vi "Init Event materiel Start.vi"(8 "error in (no error)":errorcluster caption="entrée d'erreur (pas d'erreur)", 9 "Event start test":refnum<user-event>, 10 "Part Number PCBA":string(combo), 11 "Type Product":string(combo)) -> (0 "error out":errorcluster caption="sortie d'erreur")   [LabVIEW 2020]
uses:
  Class/Instrument/Instrument (Default)/Class Instrument (Default).lvclass
  TypeDef/Variable Printable.ctl
  Class/Core/Actors/Actor_EventStart/Actor_EventStart/Actor_EventStart.lvclass
  C:/Program Files (x86)/National Instruments/LabVIEW 2020/vi.lib/ActorFramework/Actor/Actor.lvclass
  Class/Core/Actors/Actor_EventStart/Actor_EventStart Messages/Message Show_GUI/Message Show_GUI.lvclass/Message Show_GUI.ctl
  <vilib>/ActorFramework/Message Enqueuer/Message Enqueuer.lvclass/Message Enqueuer.ctl
  Class/Core/Actors/Actor_EventStart/Actor_EventStart Messages/Message Parameter/Message Parameter.lvclass/Message Parameter.ctl
  <vilib>/ActorFramework/Message Enqueuer/Enqueue.vi
  Class/Core/Actors/Actor_EventStart/Actor_EventStart Messages/Message Show_GUI/Message Show_GUI.lvclass
  C:/Program Files (x86)/National Instruments/LabVIEW 2020/vi.lib/ActorFramework/Message/Message.lvclass
  Class/Core/Actors/Actor_EventStart/Actor_EventStart Messages/Message Parameter/Message Parameter.lvclass
  <vilib>/Utility/config.llb/Read Key (String).vi
  <vilib>/ActorFramework/Message Priority Queue/Priority Enqueue.vi
  Library Commun.lvlib
  <vilib>/Utility/config.llb/NI_LVConfig.lvlib
  <vilib>/ActorFramework/Actor/Actor.lvclass
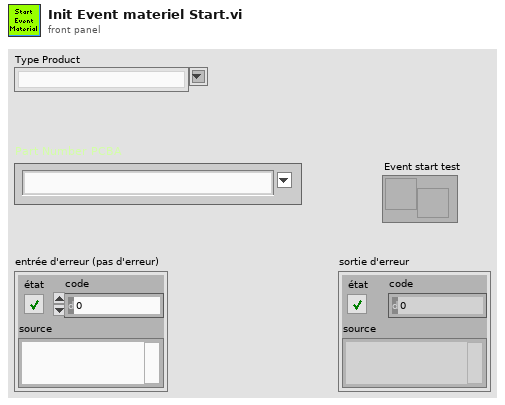
[diagram p1: front panel]
types:
  T1 = enum16{"Add Instr", "Remove Instr", "List Instr", "Get Instr Class", "Get Instr obj", "Save Insrt obj", "Modify Insrt obj", "Init"}
  T2 = enum16{"Not Use", "Wait Event", "Test in progress", "Test Stopped"}
  T3 = typedef "Variable Printable.ctl" = string
  T4 = enum16{"Get Variable", "Get All Variables", "Set Variable", "Delete Variable", "Delete All Variable"}
  T5 = cluster{"Class Event":string, "Awaited Event":string, "Instruments":refnum<class "Class Instrument (Default).lvclass">, "Event Start BP":refnum<user-event>}
  T6 = enum16{"Init", "Add Actor", "Delete Actor", "Get Actor Queue", "Get Log Actor Queue", "List all actors"}
  T7 = typedef "NI_LVConfig.lvlib/Config Data RefNum.ctl" = refnum<k1>
  T8 = cluster{"Name":string, "Instrument":refnum<class "Class Instrument (Default).lvclass">, "Close After Autotest":bool}[]
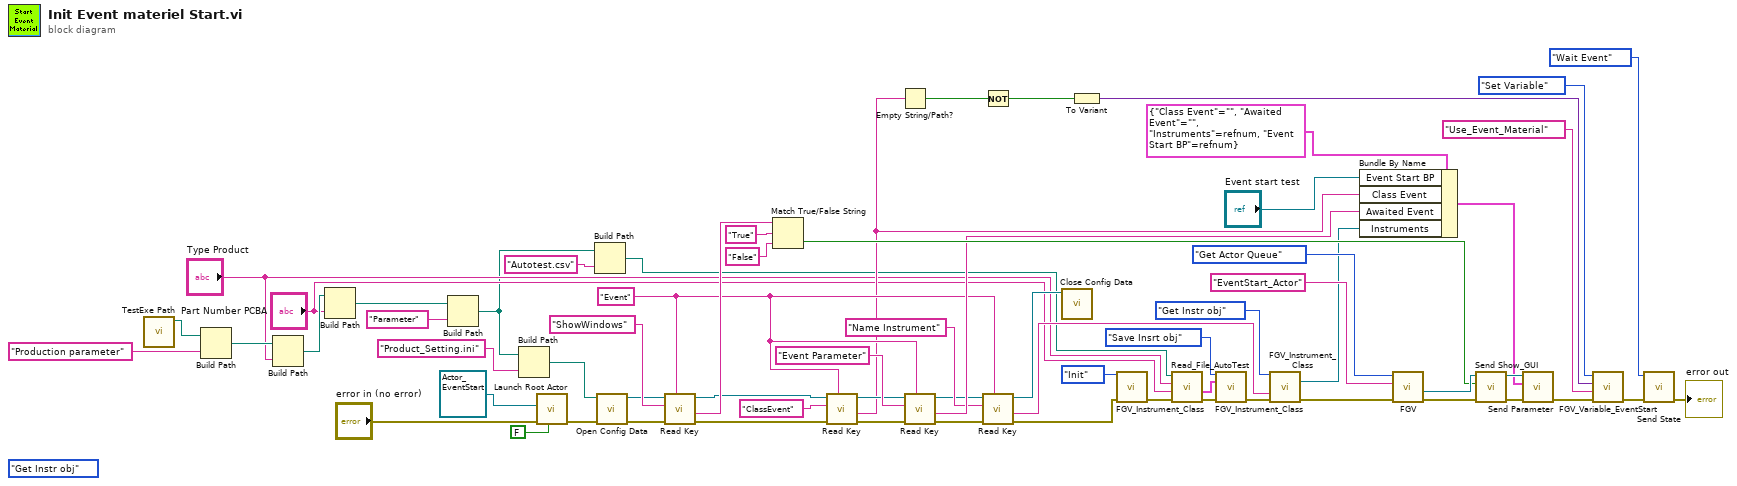
[diagram p0: block diagram]
diagram:
  (unwired) T1."Get Instr obj" ("Action")
  w39 = "Event" ("nom ou chemin relatif")
  n1 = call "TestExe Path.vi"() -> ("Chemin Actuel"=w36:path)  [unwired: 9 in, 2 out]
  n2 = Build Path(base path=w36, name or relative path="Production parameter" ("nom ou chemin relatif")) -> (appended path=w58:path)
  n3 = Build Path(base path=w58, name or relative path="Type Product") -> (appended path=w57:path)
  n4 = Build Path(base path=w57, name or relative path="Part Number PCBA") -> (appended path=w56:path)
  n5 = Build Path(base path=w56, name or relative path="Parameter" ("nom ou chemin relatif")) -> (appended path=w9:path)
  n6 = Build Path(base path=w9, name or relative path="Product_Setting.ini" ("nom ou chemin relatif")) -> (appended path=w14:path)
  n7 = call <vilib>:"Launch Root Actor.vi"("Open Actor Core front panel? (F)"=FALSE, "error in (no error)"="error in (no error)", "Actor"=refnum<class "Actor_EventStart.lvclass"> refnum ("Library Sequencer.lvlib:Actor_EventStart.lvlib:Actor_EventStart.lvclass")) -> ("error out"=w4:errorcluster)  [unwired: 7 in, 1 out]
  n8 = Build Path(base path=w9, name or relative path="Autotest.csv" ("nom ou chemin relatif")) -> (appended path=w19:path)
  n9 = call <vilib>:"Open Config Data.vi"("error in (no error)"=w4, "configuration file path"=w14) -> ("error out"=w53:errorcluster, "refnum"=w52:T7)  [unwired: 7 in, 1 out]
  n10 = call-poly <vilib>:"Read Key.vi"("section"=w39, "error in (no error)"=w53, "key"="ShowWindows", "refnum"=w52) -> ("error out"=w47:errorcluster, "value"=w49:string, "refnum out"=w31:T7)  [unwired: 4 in, 1 out]
  n11 = Match True/False String(2:"False" ("chaîne faux"), 3:"True" ("chaîne vrai"), 4:w49) -> (0:w48:bool)  [unwired: 1 out]
  n12 = call-poly <vilib>:"Read Key.vi"("section"=w39, "error in (no error)"=w47, "key"="ClassEvent", "refnum"=w31) -> ("error out"=w41:errorcluster, "value"=w25:string, "refnum out"=w30:T7)  [unwired: 4 in, 1 out]
  n13 = Empty String/Path?(string/path=w25) -> (empty?=w24:bool)
  n14 = call-poly <vilib>:"Read Key.vi"("section"=w39, "error in (no error)"=w41, "key"="Event Parameter", "refnum"=w30) -> ("error out"=w40:errorcluster, "value"=w43:string, "refnum out"=w29:T7)  [unwired: 4 in, 1 out]
  n15 = Not(x=w24) -> (.not. x?=w20:bool)
  n16 = call-poly <vilib>:"Read Key.vi"("section"=w39, "error in (no error)"=w40, "key"="Name Instrument", "refnum"=w29) -> ("error out"=w13:errorcluster, "value"=w34:string, "refnum out"=w37:T7)  [unwired: 4 in, 1 out]
  n17 = call <vilib>:"Close Config Data.vi"("refnum"=w37) -> ()  [unwired: 9 in, 2 out]
  n18 = To Variant(anything=w20) -> (Variant=w26:variant)
  n19 = call "FGV_Instrument_Class.vi"("Action"=T1."Init", "error in (no error)"=w13) -> ("error out"=w15:errorcluster)  [unwired: 11 in, 2 out]
  n20 = call "Read_File_AutoTest.vi"("error in"=w15, "Part Number PCBA"="Part Number PCBA", "Type Product"="Type Product", "file path"=w19) -> ("error out"=w16:errorcluster, "Instruments"=w17:T8)  [unwired: 4 in, 2 out]
  n21 = call "FGV_Instrument_Class.vi"("Action"=T1."Save Insrt obj", "Instruments"=w17, "error in (no error)"=w16) -> ("error out"=w12:errorcluster)  [unwired: 10 in, 2 out]
  n22 = call "FGV_Instrument_Class.vi"("Action"=T1."Get Instr obj", "Instr name"=w34, "error in (no error)"=w12) -> ("Familly class Out"=w32:refnum<class "Class Instrument (Default).lvclass">, "error out"=w33:errorcluster)  [unwired: 10 in, 1 out]
  n23 = Bundle By Name(cluster=T5 {"Class Event"="", "Awaited Event"="", "Instruments"=refnum, "Event Start BP"=refnum} ("Parameter"), "Event Start BP"="Event start test", "Class Event"=w25, "Awaited Event"=w43, "Instruments"=w32) -> (w42:T5)
  n24 = call "FGV.vi"("error in (no error)"=w33, "Actor name"="EventStart_Actor", "Action"=T6."Get Actor Queue") -> ("error out"=w62:errorcluster, "Actor's Queue Out"=w64:refnum<class "Message Enqueuer.lvclass">)  [unwired: 6 in, 1 out]
  n25 = call "Send Show_GUI.vi"("error in (no error)"=w62, "Show_GUI"=w48, "Message Enqueuer"=w64) -> ("error out"=w61:errorcluster, "Message Enqueuer out"=w63:refnum<class "Message Enqueuer.lvclass">)  [unwired: 7 in]
  n26 = call "Send Parameter.vi"("error in (no error)"=w61, "Parameter"=w42, "Message Enqueuer"=w63) -> ("error out"=w28:errorcluster)  [unwired: 7 in, 1 out]
  n27 = call "FGV_Variable_EventStart.vi"("error in (no error)"=w28, "Variable"=T3 "Use_Event_Material", "Data In"=w26, "Function"=T4."Set Variable") -> ("error out"=w22:errorcluster)  [unwired: 5 in, 2 out]
  n28 = call "Send State.vi"("entrée d'erreur (pas d'erreur)"=w22, "State"=T2."Wait Event") -> ("sortie d'erreur"=→"error out":errorcluster)  [unwired: 9 in]
